vi "rohit2Darray.vi"() -> ()   [LabVIEW 2009]
panel:
  out "Array":dbl[][](array[numeric])
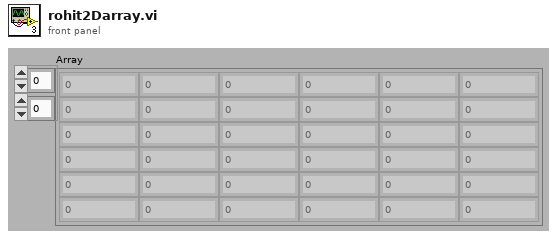
[diagram p1: front panel]
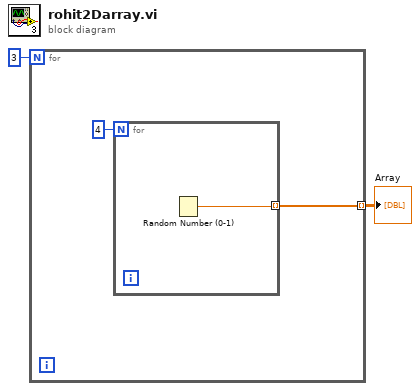
[diagram p0: block diagram]
diagram:
  n1 = for {
    N: 3 -> [_]
    tunnel: [w4] -> w1 mode=indexing
    n2 = for {
      N: 4 -> [_]
      tunnel: [w5] -> w4 mode=indexing
      n3 = Random Number (0-1)() -> (number: 0 to 1=w5:dbl)
    }
  }
  "Array" <- w1
